vi "CalcTorqueFromTension.vi"(8 "error in (no error)":errorcluster, 11 "CAlexData2 in":refnum<class "CAlex2_Data.lvclass">) -> (0 "error out":errorcluster, 1 "Joint Torque Actual":dbl[][](array[numeric]), 2 "Joint Torque Desired":dbl[][](array[numeric]), 3 "CAlexData2 out":refnum<class "CAlex2_Data.lvclass">, 4 "Tension Actual":dbl[][](array[numeric]), 6 "Tension Desired":dbl[][](array[numeric]))   [LabVIEW 2016, in "CAlex2_Data.lvclass"]
uses:
  CAlex2_Data.lvclass
  C:/Users/randh/Desktop/BILATERAL/CAlex2-controller/Sim&Process/DataProcess/ExpData/ExpData.lvclass
  CAlex2_Data.lvclass/CAlex2_Data.ctl
  Classes/CAlex2/CAlex2.lvclass
  C:/Users/randh/Desktop/BILATERAL/CAlex2-controller/Classes/SerialChain/SerialChain.lvclass
  C:/Users/randh/Desktop/BILATERAL/CAlex2-controller/Classes/SerialChain-Cable/SerialChain-Cable.lvclass
  ExpData/ExpData.lvclass
  Classes/SerialChain-Cable/SerialChain-Cable.lvclass
  Classes/SerialChain/SerialChain.lvclass
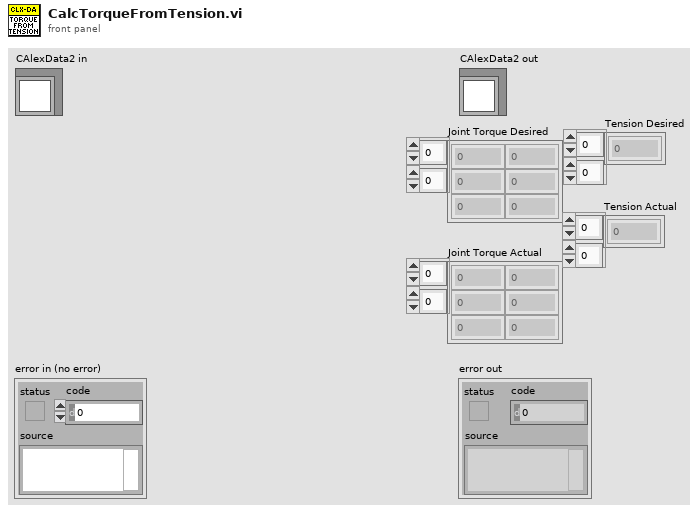
[diagram p1: front panel]
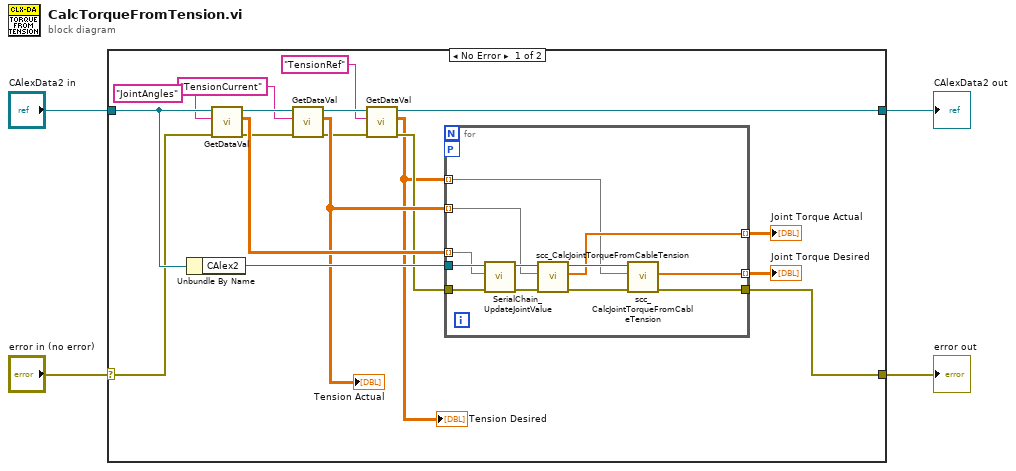
[diagram p0: block diagram]
diagram:
  n1 = case shown="No Error" "error in (no error)" {
    selector: "error in (no error)" -> [w13 w36]
    tunnel: [w12 w36] -> w3
    tunnel: [w9 w35] -> w1
    tunnel: "CAlexData2 in" -> [w21 w35]
    frame No Error {
      n2 = Unbundle By Name(w21) -> ("CAlex2"=w20:refnum<class "CAlex2.lvclass">)
      n3 = call "GetDataVal.vi"("error in (no error)"=w13, "Name"="JointAngles", "ExpData in"=w21) -> ("error out"=w14:errorcluster, "Data"=w17:dbl[][], "ExpData out"=w22:refnum<class "CAlex2_Data.lvclass">)  [unwired: 5 in, 1 out]
      n4 = call "GetDataVal.vi"("error in (no error)"=w14, "Name"="TensionCurrent", "ExpData in"=w22) -> ("error out"=w8:errorcluster, "Data"=w16:dbl[][], "ExpData out"=w10:refnum<class "CAlex2_Data.lvclass">)  [unwired: 5 in, 1 out]
      "Tension Actual" <- w16
      n5 = call "GetDataVal.vi"("error in (no error)"=w8, "Name"="TensionRef", "ExpData in"=w10) -> ("error out"=w7:errorcluster, "Data"=w6:dbl[][], "ExpData out"=w9:refnum<class "CAlex2_Data.lvclass">)  [unwired: 5 in, 1 out]
      "Tension Desired" <- w6
      n6 = for {
        tunnel: w17 -> [w33] mode=indexing
        tunnel: w16 -> [w24] mode=indexing
        tunnel: [w26] -> w15 mode=indexing
        tunnel: w20 -> [w34]
        tunnel: w7 -> [w30]
        tunnel: [w27] -> w12
        workers-P: _ -> [_]
        tunnel: [w25] -> w11 mode=indexing
        tunnel: w6 -> [w23] mode=indexing
        n7 = call "SerialChain_UpdateJointValue.vi"("error in (no error)"=w30, "JointAngle (rad | m)"=w33, "SerialChain in"=w34) -> ("error out"=w31:errorcluster, "SerialChain out"=w32:refnum<class "CAlex2.lvclass">)  [unwired: 7 in]
        n8 = call "scc_CalcJointTorqueFromCableTension.vi"("error in (no error)"=w31, "Cable Tensions"=w24, "SerialChain_Cable in"=w32) -> ("error out"=w28:errorcluster, "Joint Torque"=w25:dbl[], "SerialChain_Cable out"=w29:refnum<class "CAlex2.lvclass">)  [unwired: 5 in, 1 out]
        n9 = call "scc_CalcJointTorqueFromCableTension.vi"("error in (no error)"=w28, "Cable Tensions"=w23, "SerialChain_Cable in"=w29) -> ("error out"=w27:errorcluster, "Joint Torque"=w26:dbl[])  [unwired: 5 in, 2 out]
      }
      "Joint Torque Desired" <- w15
      "Joint Torque Actual" <- w11
    }
    frame Error {
    }
  }
  "error out" <- w3
  "CAlexData2 out" <- w1
